vi "Main.vi"(8 "error in":errorcluster, 11 "Message Pump Tester":refnum<class "Message Pump Tester.lvclass">) -> (0 "error out":errorcluster, 3 "Message Pump Tester out":refnum<class "Message Pump Tester.lvclass">)   [LabVIEW 2017, in "Message Pump Tester.lvclass"]
doc: "The <b>Queued Message Handler</b> of the Worker that owns this VI."
uses:
  Message Pump Tester.lvclass
  C:/SC/Source Code/VIPM/LabVIEW 20xx/vi.lib/addons/_Workers/Library/Classes/Worker/Worker.lvclass
  <vilib>/addons/_Workers/Library/Classes/Message Queue/Message Queue.lvclass
  Message Pump/_Message Pump.lvclass
panel:
  in  "Stop":bool
  in  "Start":bool
  out "Value":u32
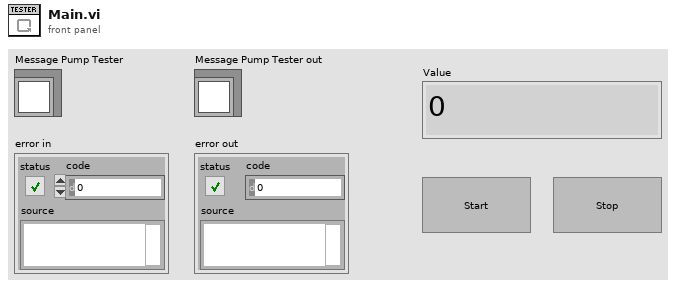
[diagram p1: front panel]
types:
  T1 = typedef "Workers.lvlib/Case Label.ctl" = string
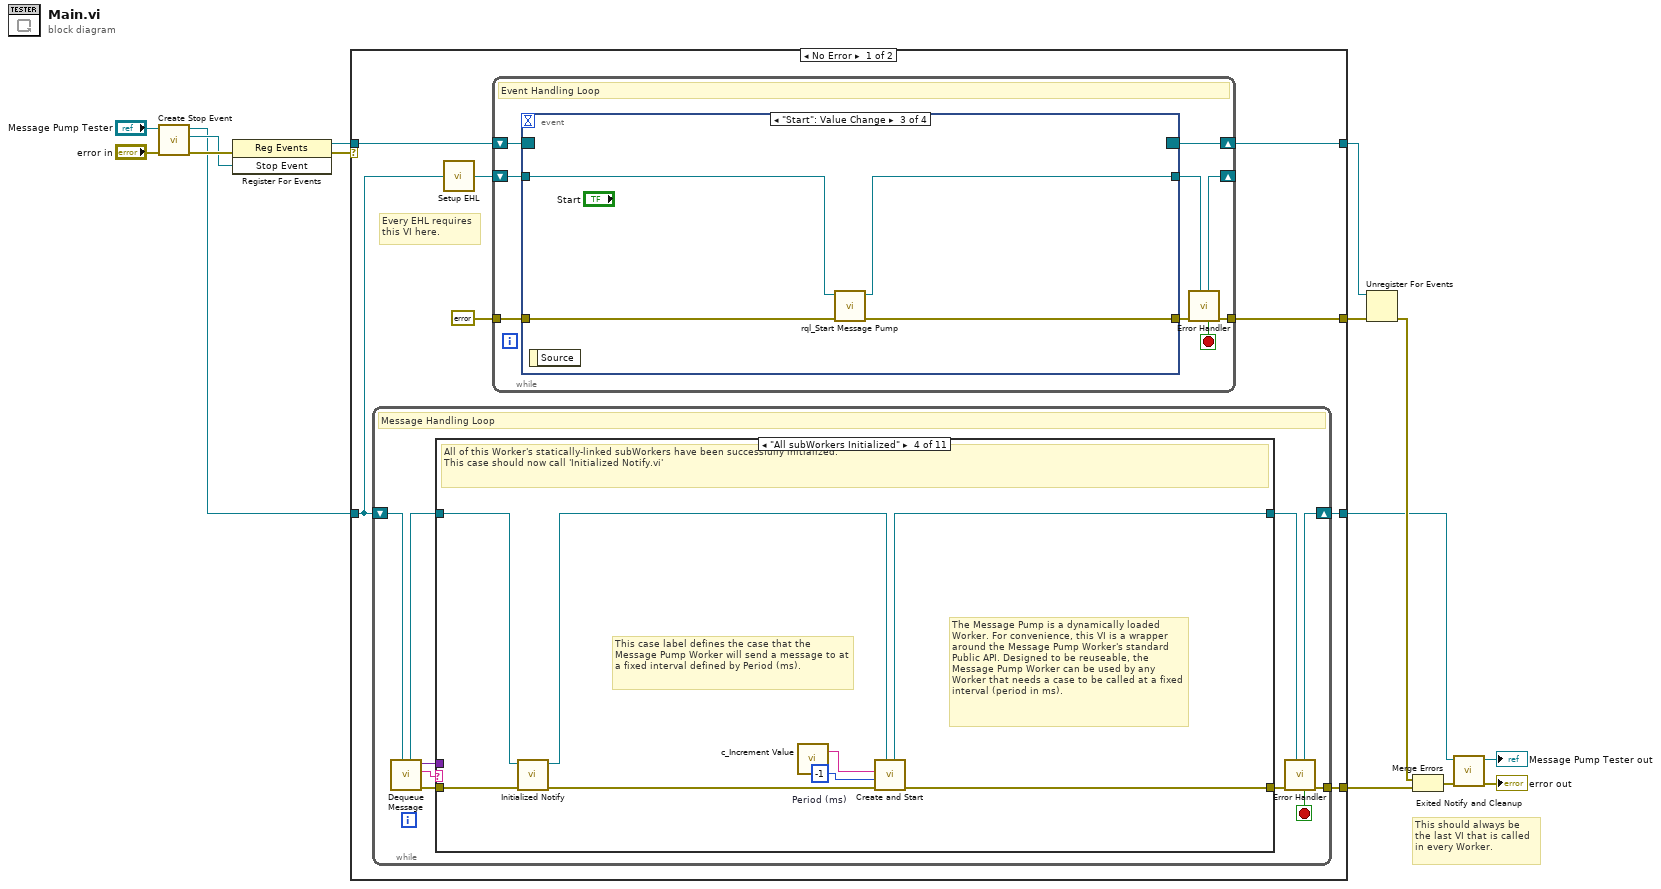
[diagram p0: block diagram]
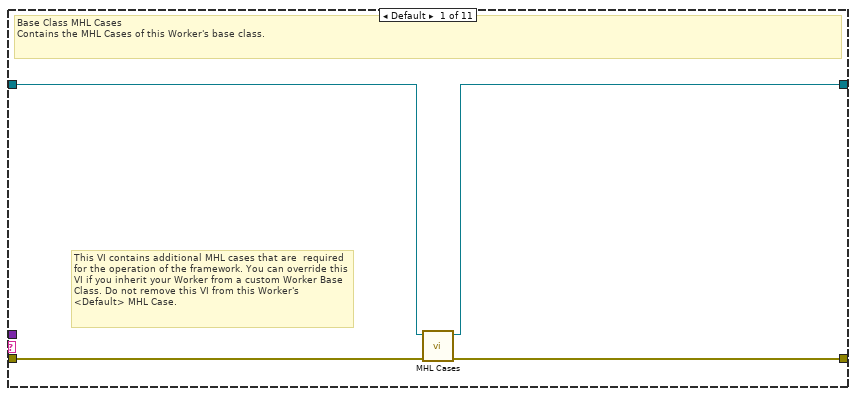
[diagram p2: hidden frame]
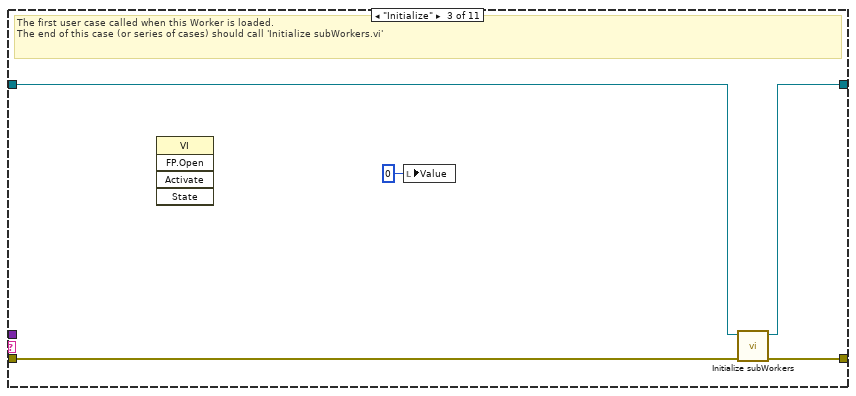
[diagram p4: hidden frame]
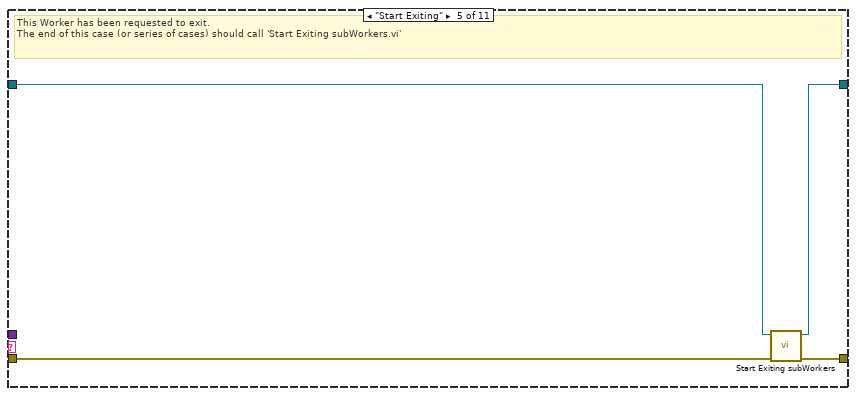
[diagram p5: hidden frame]
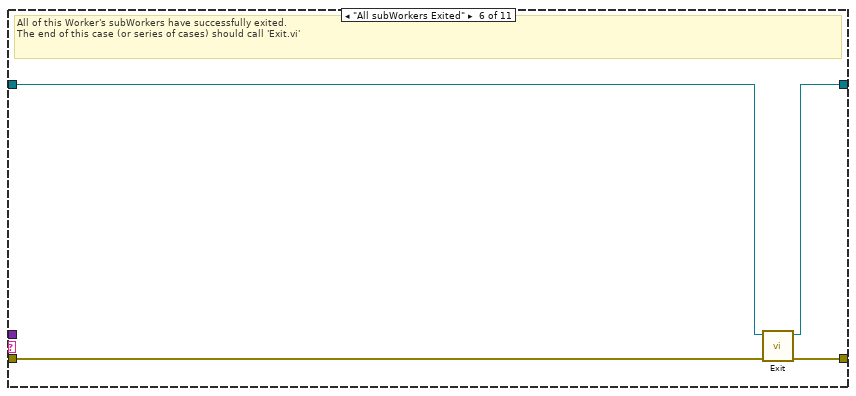
[diagram p6: hidden frame]
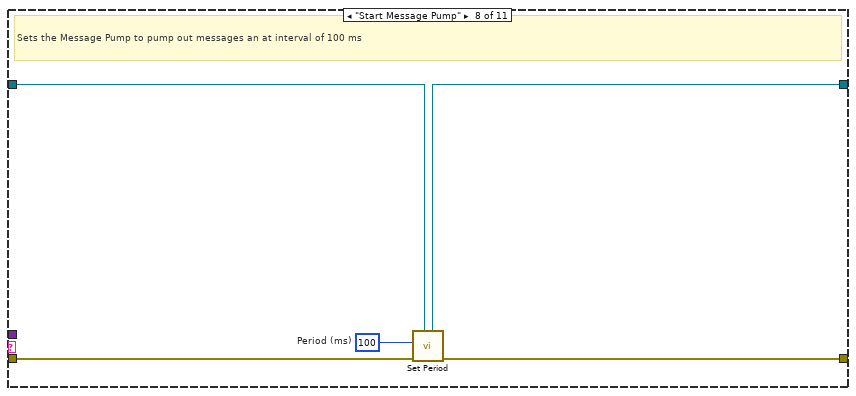
[diagram p8: hidden frame]
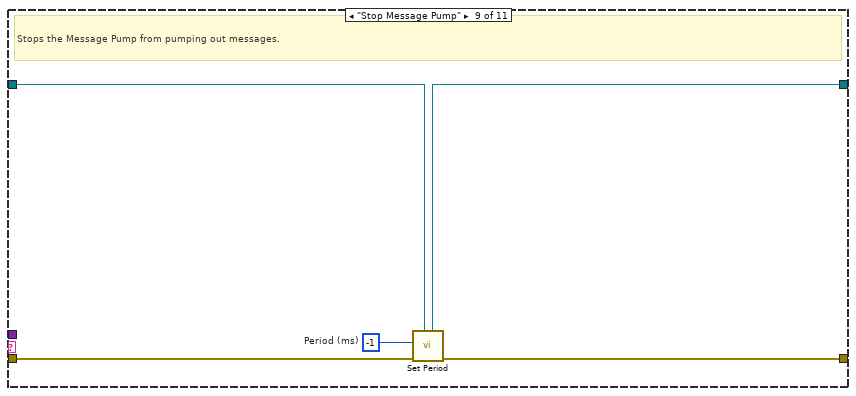
[diagram p9: hidden frame]
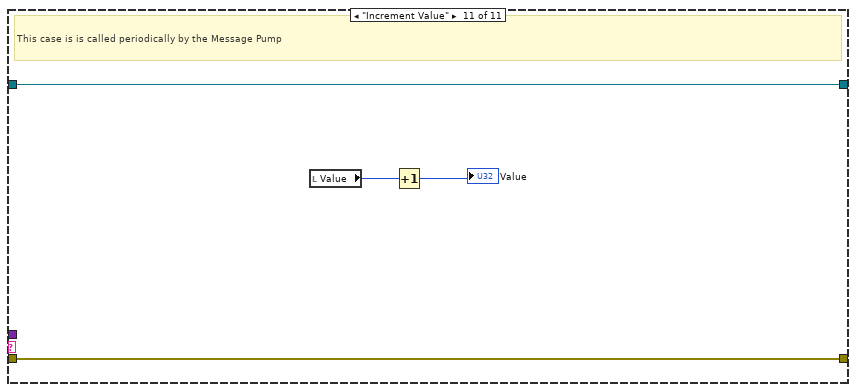
[diagram p11: hidden frame]
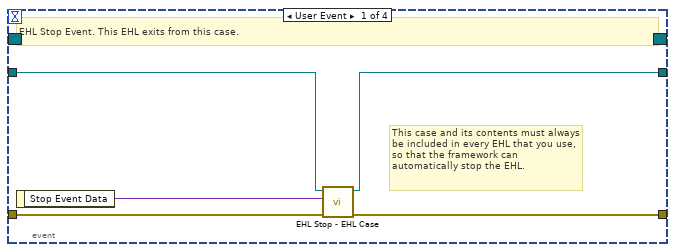
[diagram p12: hidden frame]
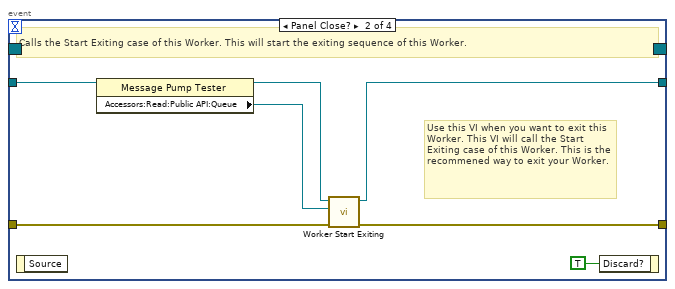
[diagram p13: hidden frame]
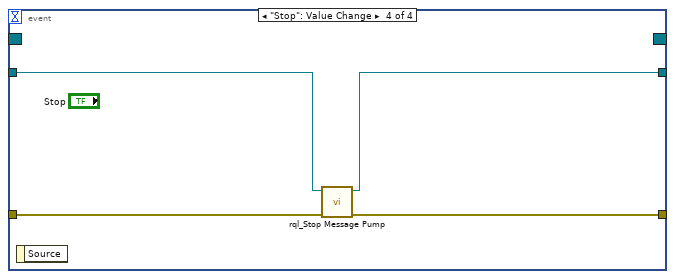
[diagram p14: hidden frame]
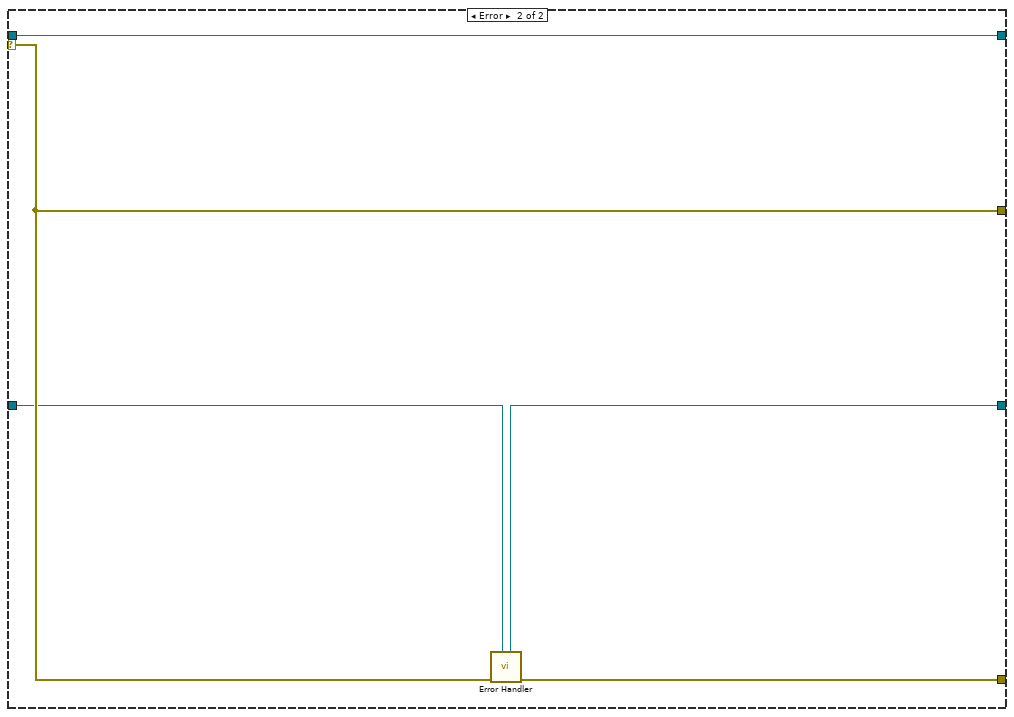
[diagram p15: hidden frame]
diagram:
  # "This should always be the last VI that is called in every Worker."
  n1 = call-dynamic "Create Stop Event.vi"("error in"="error in", "Worker"="Message Pump Tester") -> ("error out"=w10:errorcluster, "Stop Event"=w7:refnum<user-event>, "Worker out"=w4:refnum<class "Message Pump Tester.lvclass">)  [unwired: 7 in]
  n2 = register-events(error in=w10, w7) -> (reference out=w9:refnum<event-registration>, error out=w1:errorcluster)  [unwired: 1 in]
  n3 = case shown="No Error" w1 {
    tunnel: w4 -> [w18 w109]
    tunnel: [w16 w110] -> w8
    tunnel: w9 -> [w23 w111]
    tunnel: [w20 w112] -> w14
    tunnel: [w22 w111] -> w13
    tunnel: [w17 w108] -> w11
    selector: w1 -> [_ w112]
    frame No Error {
      # "Every EHL requires\nthis VI here."
      n4 = while {
        shift-right: [w31] -> w17
        shift-left: w18 -> [w33]
        tunnel: [w32] -> w16
        stop <- w25 stop-if-true
        # "Message Handling Loop"
        n5 = call-dynamic "Dequeue Message.vi"("Worker"=w33) -> ("error out"=w30:errorcluster, "Case out"=w26:string, "Data out"=w24:variant, "Worker out"=w28:refnum<class "Message Pump Tester.lvclass">)  [unwired: 6 in, 1 out]
        n6 = case "Worker MHL Case Structure (DO NOT CHANGE LABEL NAME)" shown="\"All subWorkers Initialized\"" w26 {
          tunnel: w30 -> [w37 w38 w42 w51 w53 w60 w62 w67 w72 w74 w78]
          tunnel: [w36 w38 w44 w49 w56 w59 w62 w66 w71 w74 w78] -> w29
          tunnel: w28 -> [w35 w39 w41 w52 w54 w58 w61 w64 w69 w73 w77]
          tunnel: [w34 w39 w43 w45 w55 w57 w61 w63 w68 w73 w77] -> w27
          tunnel: w24 -> [_ _ _ _ _ _ _ _ _ _ _]
          frame Default {
            # "This VI contains additional MHL cases that are  required for the operation of the framework. You can override this VI if you inherit your Worker from a custom Worker Base Class. Do not remove this VI from this Worker's <Default> MHL Case."
            # "Base Class MHL Cases\nContains the MHL Cases of this Worker's base class."
            n7 = call-dynamic "MHL Cases.vi"("error in"=w37, "Worker in"=w35) -> ("error out"=w36:errorcluster, "Worker out"=w34:refnum<class "Message Pump Tester.lvclass">)  [unwired: 8 in]
          }
          frame "------------ FRAMEWORK CASES -----------" {
            # "Start of Workers Framework Cases"
          }
          frame "Initialize" {
            # "The first user case called when this Worker is loaded.\nThe end of this case (or series of cases) should call 'Initialize subWorkers.vi'"
            n8 = invoke class="VI" method="FP.Open"() -> ()  [unwired: 5 in, 5 out]
            n9 = local write "Value"(u32 0 ("Value")) -> ()
            n10 = call-dynamic "Initialize subWorkers.vi"("error in"=w42, "Worker"=w41) -> ("error out"=w44:errorcluster, "dup Worker out"=w43:refnum<class "Message Pump Tester.lvclass">)  [unwired: 8 in]
          }
          frame "All subWorkers Initialized" {
            w50 = -1  # Period (ms)
            # "This case label defines the case that the Message Pump Worker will send a message to at a fixed interval defined by Period (ms)."
            # "The Message Pump is a dynamically loaded Worker. For convenience, this VI is a wrapper around the Message Pump Worker's standard Public API. Designed to be reuseable, the Message Pump Worker can be used by any Worker that needs a case to be called at a fixed interval (period in ms)."
            # "All of this Worker's statically-linked subWorkers have been successfully initialized.\nThis case should now call 'Initialized Notify.vi'"
            n11 = call-dynamic "Initialized Notify.vi"("error in"=w51, "Worker"=w52) -> ("error out"=w47:errorcluster, "dup Worker out"=w46:refnum<class "Message Pump Tester.lvclass">)  [unwired: 8 in]
            n12 = call "c_Increment Value.vi"() -> ("Case Label"=w48:T1)  [unwired: 1 in]
            n13 = call "Create and Start.vi"("Caller"=w46, "error in (no error)"=w47, "Period (ms)"=w50, "Time Elapsed Response Case (Case Label)"=w48) -> ("error out"=w49:errorcluster, "dup Caller out"=w45:refnum<class "Message Pump Tester.lvclass">)  [unwired: 5 in, 1 out]
          }
          frame "Start Exiting" {
            # "This Worker has been requested to exit. \nThe end of this case (or series of cases) should call 'Start Exiting subWorkers.vi'"
            n14 = call-dynamic "Start Exiting subWorkers.vi"("error_in"=w53, "Worker"=w54) -> ("error out"=w56:errorcluster, "dup Worker out"=w55:refnum<class "Message Pump Tester.lvclass">)  [unwired: 8 in]
          }
          frame "All subWorkers Exited" {
            # "All of this Worker's subWorkers have successfully exited. \nThe end of this case (or series of cases) should call 'Exit.vi'"
            n15 = call-dynamic "Exit.vi"("error_in"=w60, "Worker"=w58) -> ("error out"=w59:errorcluster, "dup Worker out"=w57:refnum<class "Message Pump Tester.lvclass">)  [unwired: 8 in]
          }
          frame "------------- LOCAL API CASES -------------" {
            # "Start of Workers Local API Cases"
          }
          frame "Start Message Pump" {
            w65 = 100  # Period (ms)
            # "Sets the Message Pump to pump out messages an at interval of 100 ms"
            n16 = call "Set Period.vi"("Caller"=w64, "error in"=w67, "Period (ms)"=w65) -> ("error out"=w66:errorcluster, "dup Caller out"=w63:refnum<class "Message Pump Tester.lvclass">)  [unwired: 7 in]
          }
          frame "Stop Message Pump" {
            w70 = -1  # Period (ms)
            # "Stops the Message Pump from pumping out messages."
            n17 = call "Set Period.vi"("Caller"=w69, "error in"=w72, "Period (ms)"=w70) -> ("error out"=w71:errorcluster, "dup Caller out"=w68:refnum<class "Message Pump Tester.lvclass">)  [unwired: 7 in]
          }
          frame "------------- RESPONSE CASES --------------" {
            # "Start of Workers Response Cases"
          }
          frame "Increment Value" {
            # "This case is is called periodically by the Message Pump"
            n18 = local read "Value"() -> (w76:u32)
            n19 = Increment(x=w76) -> (x+1=→"Value":u32)
          }
        }
        n20 = call-dynamic "Error Handler.vi"("Worker"=w27, "error_in"=w29) -> ("error out"=w32:errorcluster, "Stop Loop"=w25:bool, "Worker out"=w31:refnum<class "Message Pump Tester.lvclass">)  [unwired: 7 in]
      }
      n21 = call-dynamic "Setup EHL.vi"("Worker"=w18) -> ("Worker out"=w19:refnum<class "Message Pump Tester.lvclass">)  [unwired: 14 in]
      n22 = while "Event Handling Loop" {
        shift-right: [w87] -> w22
        shift-left: w23 -> [w86]
        tunnel: [w82] -> w20
        tunnel: errorcluster {"status"=FALSE, "code"=0, "source"=""} ("error constant") -> [w84]
        shift-right: [w80] -> _
        shift-left: w19 -> [w85]
        stop <- w79 stop-if-true
        # "Event Handling Loop"
        n23 = event shown="[2] \"Start\": Value Change" {
          selector: w86 -> [_ _ _ _]
          dyn-events: [_ _ _ _] -> w87
          timeout: _ -> [_ _ _ _]
          tunnel: [w91 w98 w102 w106] -> w83
          tunnel: w84 -> [w92 w97 w103 w107]
          tunnel: w85 -> [w90 w96 w101 w105]
          tunnel: [w89 w95 w100 w104] -> w81
          event User Event {
            # "This case and its contents must always be included in every EHL that you use, so that the framework can automatically stop the EHL."
            # "EHL Stop Event. This EHL exits from this case."
            n24 = event-data() -> ("Stop Event Data"=w88:variant)  [unwired: 1 in]
            n25 = call-dynamic "EHL Stop - EHL Case.vi"("error in"=w92, "Stop Event Data"=w88, "Worker"=w90) -> ("error out"=w91:errorcluster, "Worker out"=w89:refnum<class "Message Pump Tester.lvclass">)  [unwired: 7 in]
          }
          event Panel Close? {
            # "Use this VI when you want to exit this Worker. This VI will call the Start Exiting case of this Worker. This is the recommened way to exit your Worker."
            # "Calls the Start Exiting case of this Worker. This will start the exiting sequence of this Worker."
            n26 = event-data() -> ()  [unwired: 1 in, 1 out]
            n27 = property class="Message Pump Tester"(reference=w96) -> (reference out=w94:refnum<class "Message Pump Tester.lvclass">, "Accessors:Read:Public API:Queue"=w93:refnum<class "Message Queue.lvclass">)  [unwired: 1 in, 1 out]
            n28 = call-dynamic "Worker Start Exiting.vi"("error_in"=w97, "Message Queue"=w93, "Worker"=w94) -> ("error out"=w98:errorcluster, "dup Worker out"=w95:refnum<class "Message Pump Tester.lvclass">)  [unwired: 7 in]
            n29 = event-data("Discard?"=TRUE) -> ()  [unwired: 1 in, 1 out]
          }
          event "Start": Value Change {
            n30 = event-data() -> ()  [unwired: 1 in, 1 out]
            n31 = call "rql_Start Message Pump.vi"("error in"=w103, "Message Pump Tester in"=w101) -> ("error out"=w102:errorcluster, "dup Message Pump Tester out"=w100:refnum<class "Message Pump Tester.lvclass">)  [unwired: 8 in]
          }
          event "Stop": Value Change {
            n32 = event-data() -> ()  [unwired: 1 in, 1 out]
            n33 = call "rql_Stop Message Pump.vi"("error in"=w107, "Message Pump Tester in"=w105) -> ("error out"=w106:errorcluster, "dup Message Pump Tester out"=w104:refnum<class "Message Pump Tester.lvclass">)  [unwired: 8 in]
          }
        }
        n34 = call-dynamic "Error Handler.vi"("Worker"=w81, "error_in"=w83) -> ("error out"=w82:errorcluster, "Stop Loop"=w79:bool, "Worker out"=w80:refnum<class "Message Pump Tester.lvclass">)  [unwired: 7 in]
      }
    }
    frame Error {
      n35 = call-dynamic "Error Handler.vi"("Worker"=w109, "error_in"=w112) -> ("error out"=w110:errorcluster, "Worker out"=w108:refnum<class "Message Pump Tester.lvclass">)  [unwired: 7 in, 1 out]
    }
  }
  n36 = Unregister For Events(event registration refnum=w13, error in=w14) -> (error out=w15:errorcluster)
  n37 = Merge Errors(w15, w8) -> (w12:errorcluster)
  n38 = call-dynamic "Exited Notify and Cleanup.vi"("error_in"=w12, "Worker"=w11) -> ("error out"=→"error out":errorcluster, "dup Worker out"=→"Message Pump Tester out":refnum<class "Message Pump Tester.lvclass">)  [unwired: 8 in]
